vi "DB- read write.vi"(4 "cmd":string="Where ENGINE='", 5 "database cluster write data in":T1={"ID"=0, "Datetime"="17-03-2020 14:45:50", "PARTBARCODE"="", "TORQUE"="", "RESULT1"="", "CHILD1"="", "CHILD2"="A1234567B567003", "CHILD3"="", "CHILD4"="", "RESULT2"="OK", "FINALBARCODE"="", "RESULT3"="", "REMARK"="", "OTHER"=""}, 6 "action":T3(ring), 8 "error in (no error)":errorcluster, 9 "cloumns":string[](array[string]), 10 "BARCODE":string, 11 "connection reference":T2) -> (0 "error out":errorcluster, 1 "Dispalya":string[](array[string]), 2 "Data Read":variant[][](array[variant]), 3 "Refnum out":T2)   [LabVIEW 2023]
uses:
  <vilib>/addons/database/Connection.llb/Conn ObjectReference.ctl
  database cluster.ctl
  <vilib>/addons/database/NI_Database_API.lvlib
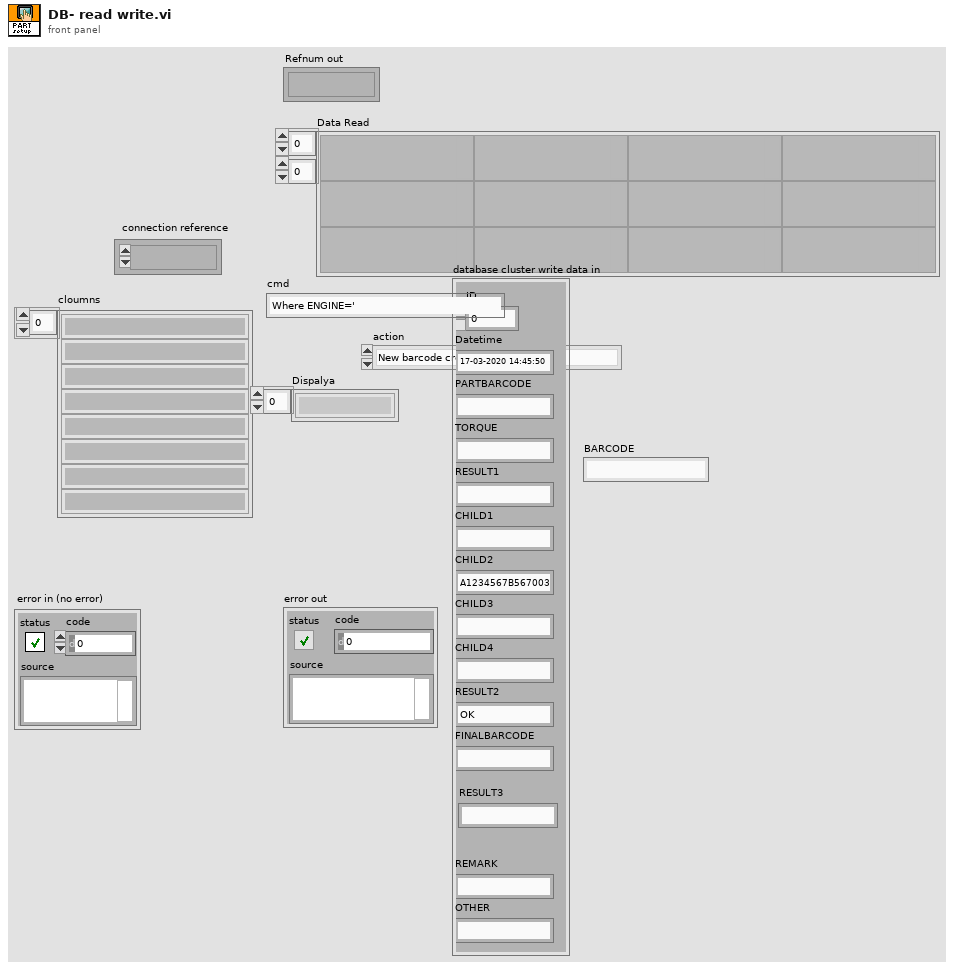
[diagram p1: front panel]
types:
  T1 = typedef "database cluster.ctl" = cluster{"ID":i64, "Datetime":string, "PARTBARCODE":string, "TORQUE":string, "RESULT1":string, "CHILD1":string, "CHILD2":string, "CHILD3":string, "CHILD4":string, "RESULT2":string, "FINALBARCODE":string, "RESULT3":string, "REMARK":string, "OTHER":string}
  T2 = typedef "NI_Database_API.lvlib/Conn ObjectReference.ctl" = refnum<k1>
  T3 = enum16{"New barcode create", "barcode update", "check barcode", "database read", "barcode delete"}
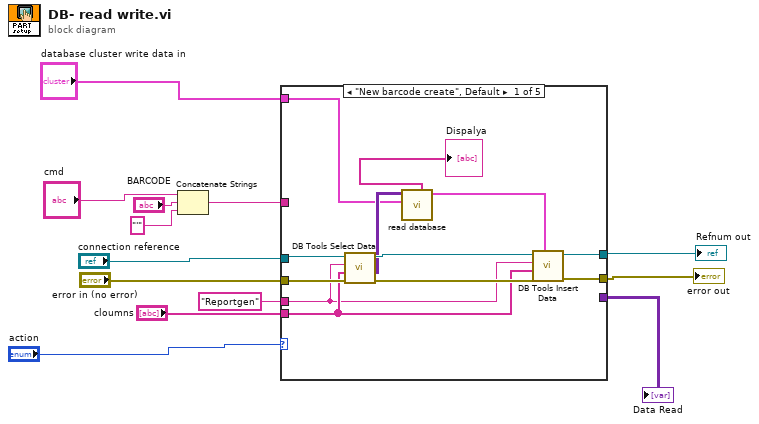
[diagram p0: block diagram]
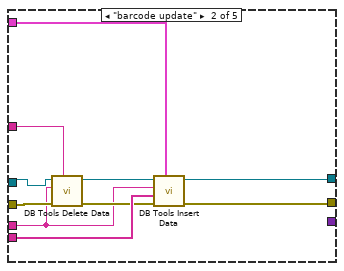
[diagram p2: hidden frame]
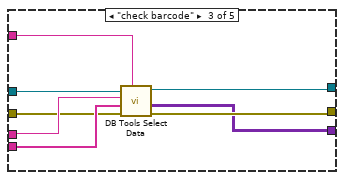
[diagram p3: hidden frame]
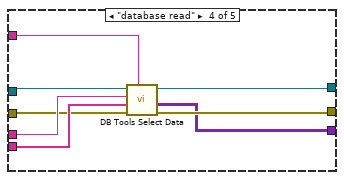
[diagram p4: hidden frame]
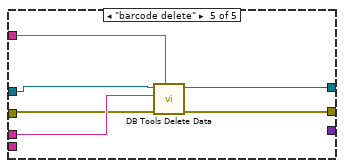
[diagram p5: hidden frame]
diagram:
  n1 = Concatenate Strings("cmd", "BARCODE", "'" ("string")) -> (w10:string)
  n2 = case shown="\"New barcode create\", Default" "action" {
    tunnel: [w25 w35 w40 w51 w57] -> w5
    tunnel: [w24 w34 w39 w50 w56] -> w6
    tunnel: w10 -> [_ w28 w43 w44 w55]
    tunnel: "cloumns" -> [w17 w33 w42 w47 _]
    tunnel: "Reportgen" ("table") -> [w16 w27 w41 w48 w54]
    tunnel: [_ _ w38 w49 _] -> w13
    tunnel: "connection reference" -> [w23 w32 w37 w46 w53]
    tunnel: "error in (no error)" -> [w22 w29 w36 w45 w52]
    tunnel: "database cluster write data in" -> [w15 w26 _ _ _]
    frame "New barcode create", Default {
      n3 = call <vilib>:"DB Tools Select Data.vi"("error in (no error)"=w22, "columns"=w17, "table"=w16, "connection reference"=w23) -> ("error out"=w21:errorcluster, "data"=w19:variant[][], "connection reference out"=w20:T2)  [unwired: 2 in]
      n4 = call "read database.vi"("database cluster write data in 3"=w15, "Data Read"=w19) -> ("database cluster write data"=w18:T1, "Dispalya"=→"Dispalya":string[])  [unwired: 4 in, 4 out]
      n5 = call <vilib>:"DB Tools Insert Data.vi"("data"=w18, "error in (no error)"=w21, "columns"=w17, "table"=w16, "connection reference"=w20) -> ("error out"=w24:errorcluster, "connection reference out"=w25:T2)  [unwired: 5 in]
    }
    frame "barcode update" {
      n6 = call <vilib>:"DB Tools Delete Data.vi"("condition"=w28, "error in (no error)"=w29, "table"=w27, "connection reference"=w32) -> ("error out"=w30:errorcluster, "connection reference out"=w31:T2)  [unwired: 6 in]
      n7 = call <vilib>:"DB Tools Insert Data.vi"("data"=w26, "error in (no error)"=w30, "columns"=w33, "table"=w27, "connection reference"=w31) -> ("error out"=w34:errorcluster, "connection reference out"=w35:T2)  [unwired: 5 in]
    }
    frame "check barcode" {
      n8 = call <vilib>:"DB Tools Select Data.vi"("condition"=w43, "error in (no error)"=w36, "columns"=w42, "table"=w41, "connection reference"=w37) -> ("error out"=w39:errorcluster, "data"=w38:variant[][], "connection reference out"=w40:T2)  [unwired: 1 in]
    }
    frame "database read" {
      n9 = call <vilib>:"DB Tools Select Data.vi"("condition"=w44, "error in (no error)"=w45, "columns"=w47, "table"=w48, "connection reference"=w46) -> ("error out"=w50:errorcluster, "data"=w49:variant[][], "connection reference out"=w51:T2)  [unwired: 1 in]
    }
    frame "barcode delete" {
      n10 = call <vilib>:"DB Tools Delete Data.vi"("condition"=w55, "error in (no error)"=w52, "table"=w54, "connection reference"=w53) -> ("error out"=w56:errorcluster, "connection reference out"=w57:T2)  [unwired: 6 in]
    }
  }
  "Refnum out" <- w5
  "error out" <- w6
  "Data Read" <- w13
